vi "edittest write fields to file.vi"(8 "error in (no error)":errorcluster, 10 "Sequence Fields":T1[](array[typedef]), 11 "File Refnum In":T4) -> (0 "error out":errorcluster, 3 "File Refnum Out":T4)   [LabVIEW 2011]
uses:
  <vilib>/Utility/config.llb/Config Data RefNum.ctl
  server/database/Fields/Field Record.ctl
  server/database/Fields/Field DataTypes.ctl
  server/database/Fields/Field NextItem.ctl
  <vilib>/Utility/config.llb/Write Key (I32).vi
  <vilib>/Utility/config.llb/Write Key (String).vi
  <vilib>/Utility/config.llb/Write Key (Boolean).vi
  <vilib>/Utility/config.llb/NI_LVConfig.lvlib
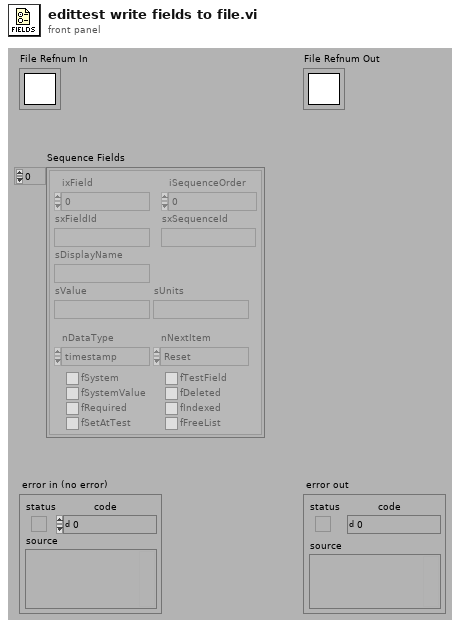
[diagram p1: front panel]
types:
  T1 = typedef "Field Record.ctl" = cluster{"ixField":i32, "iSequenceOrder":i32, "sxFieldId":string, "sxSequenceId":string, "sDisplayName":string, "sValue":string, "sUnits":string, "nDataType":T2, "nNextItem":T3, "fSystem":bool, "fSystemValue":bool, "fRequired":bool, "fSetAtTest":bool, "fTestField":bool, "fDeleted":bool, "fIndexed":bool, "fFreeList":bool}
  T2 = typedef "Field DataTypes.ctl" = enum32{"text", "numeric", "list", "timestamp", "boolean"}
  T3 = typedef "Field NextItem.ctl" = enum32{"Reset", "Retain", "Auto-Increment"}
  T4 = typedef "NI_LVConfig.lvlib/Config Data RefNum.ctl" = refnum<k1>
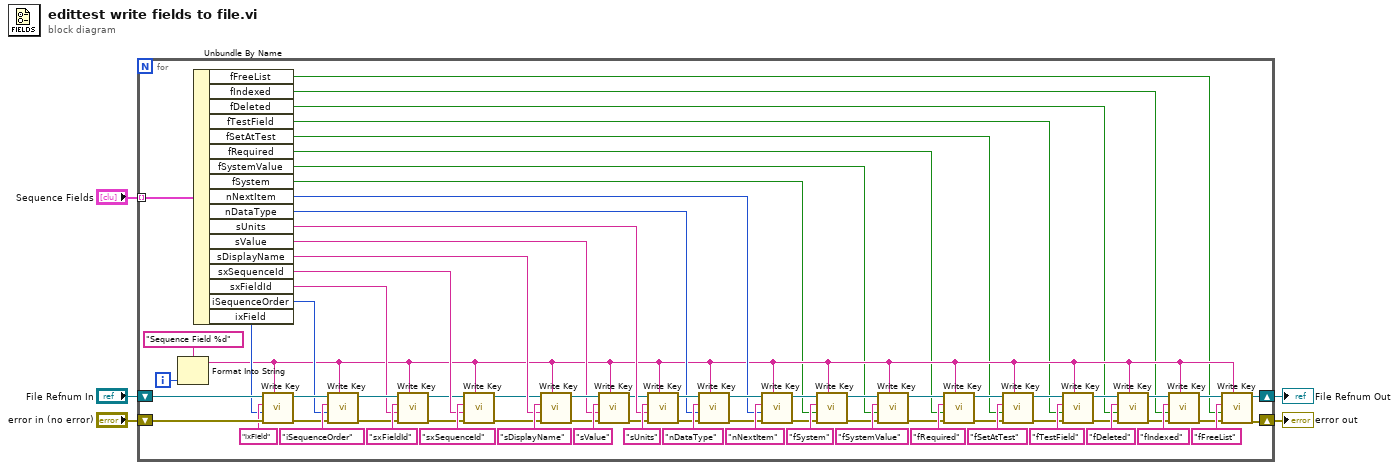
[diagram p0: block diagram]
diagram:
  n1 = for {
    shift-right: [w7] -> w4
    shift-left: "File Refnum In" -> [w75]
    shift-right: [w6] -> w5
    shift-left: "error in (no error)" -> [w76]
    tunnel: "Sequence Fields" -> [w77] mode=indexing
    i -> [w78]
    n2 = Format Into String(format string="Sequence Field %d", w78) -> (resulting string=w21:string)  [unwired: 2 in, 1 out]
    n3 = Unbundle By Name(w77) -> ("fFreeList"=w8:bool, "fIndexed"=w9:bool, "fDeleted"=w10:bool, "fTestField"=w11:bool, "fSetAtTest"=w12:bool, "fRequired"=w13:bool, "fSystemValue"=w14:bool, "fSystem"=w15:bool, "nNextItem"=w27:T3, "nDataType"=w28:T2, "sUnits"=w36:string, "sValue"=w37:string, "sDisplayName"=w42:string, "sxSequenceId"=w43:string, "sxFieldId"=w44:string, "iSequenceOrder"=w45:i32, "ixField"=w48:i32)
    n4 = call-poly <vilib>:"Write Key.vi"("section"=w21, "error in (no error)"=w76, "value"=w48, "key"="ixField", "refnum"=w75) -> ("error out"=w67:errorcluster, "refnum out"=w60:T4)  [unwired: 5 out]
    n5 = call-poly <vilib>:"Write Key.vi"("section"=w21, "error in (no error)"=w67, "value"=w45, "key"="iSequenceOrder", "refnum"=w60) -> ("error out"=w66:errorcluster, "refnum out"=w61:T4)  [unwired: 5 out]
    n6 = call-poly <vilib>:"Write Key.vi"("section"=w21, "error in (no error)"=w66, "value"=w44, "key"="sxFieldId", "refnum"=w61) -> ("error out"=w39:errorcluster, "refnum out"=w40:T4)  [unwired: 1 in, 4 out]
    n7 = call-poly <vilib>:"Write Key.vi"("section"=w21, "error in (no error)"=w39, "value"=w43, "key"="sxSequenceId", "refnum"=w40) -> ("error out"=w38:errorcluster, "refnum out"=w41:T4)  [unwired: 1 in, 4 out]
    n8 = call-poly <vilib>:"Write Key.vi"("section"=w21, "error in (no error)"=w38, "value"=w42, "key"="sDisplayName", "refnum"=w41) -> ("error out"=w58:errorcluster, "refnum out"=w57:T4)  [unwired: 1 in, 4 out]
    n9 = call-poly <vilib>:"Write Key.vi"("section"=w21, "error in (no error)"=w58, "value"=w37, "key"="sValue", "refnum"=w57) -> ("error out"=w34:errorcluster, "refnum out"=w35:T4)  [unwired: 1 in, 4 out]
    n10 = call-poly <vilib>:"Write Key.vi"("section"=w21, "error in (no error)"=w34, "value"=w36, "key"="sUnits", "refnum"=w35) -> ("error out"=w30:errorcluster, "refnum out"=w32:T4)  [unwired: 1 in, 4 out]
    n11 = call-poly <vilib>:"Write Key.vi"("section"=w21, "error in (no error)"=w30, "value"=w28, "key"="nDataType", "refnum"=w32) -> ("error out"=w29:errorcluster, "refnum out"=w31:T4)  [unwired: 5 out]
    n12 = call-poly <vilib>:"Write Key.vi"("section"=w21, "error in (no error)"=w29, "value"=w27, "key"="nNextItem", "refnum"=w31) -> ("error out"=w17:errorcluster, "refnum out"=w16:T4)  [unwired: 5 out]
    n13 = call-poly <vilib>:"Write Key.vi"("section"=w21, "error in (no error)"=w17, "value"=w15, "key"="fSystem", "refnum"=w16) -> ("error out"=w65:errorcluster, "refnum out"=w62:T4)  [unwired: 5 out]
    n14 = call-poly <vilib>:"Write Key.vi"("section"=w21, "error in (no error)"=w65, "value"=w14, "key"="fSystemValue", "refnum"=w62) -> ("error out"=w64:errorcluster, "refnum out"=w63:T4)  [unwired: 5 out]
    n15 = call-poly <vilib>:"Write Key.vi"("section"=w21, "error in (no error)"=w64, "value"=w13, "key"="fRequired", "refnum"=w63) -> ("error out"=w49:errorcluster, "refnum out"=w52:T4)  [unwired: 5 out]
    n16 = call-poly <vilib>:"Write Key.vi"("section"=w21, "error in (no error)"=w49, "value"=w12, "key"="fSetAtTest", "refnum"=w52) -> ("error out"=w50:errorcluster, "refnum out"=w51:T4)  [unwired: 5 out]
    n17 = call-poly <vilib>:"Write Key.vi"("section"=w21, "error in (no error)"=w50, "value"=w11, "key"="fTestField", "refnum"=w51) -> ("error out"=w18:errorcluster, "refnum out"=w24:T4)  [unwired: 5 out]
    n18 = call-poly <vilib>:"Write Key.vi"("section"=w21, "error in (no error)"=w18, "value"=w10, "key"="fDeleted", "refnum"=w24) -> ("error out"=w19:errorcluster, "refnum out"=w23:T4)  [unwired: 5 out]
    n19 = call-poly <vilib>:"Write Key.vi"("section"=w21, "error in (no error)"=w19, "value"=w9, "key"="fIndexed", "refnum"=w23) -> ("error out"=w20:errorcluster, "refnum out"=w22:T4)  [unwired: 5 out]
    n20 = call-poly <vilib>:"Write Key.vi"("section"=w21, "error in (no error)"=w20, "value"=w8, "key"="fFreeList", "refnum"=w22) -> ("error out"=w6:errorcluster, "refnum out"=w7:T4)  [unwired: 5 out]
  }
  "error out" <- w5
  "File Refnum Out" <- w4
